vi "WS_Main.vi"(6 "LabVIEW Web Service":refnum<class "Web Service.lvclass">) -> ()   [LabVIEW 2020]
uses:
  <vilib>/wsapi/Web Service.lvclass
  <vilib>/Utility/error.llb/DialogType.ctl
  Libraries/WSsupport/GV_Repos.vi
  Libraries/WSsupport/WSsupport.lvlib
  Libraries/Packages/VIPM/VIPM.lvlib
  Libraries/Packages/GPM/GPM.lvlib
  Libraries/Packages/Packages.lvlib
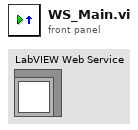
[diagram p1: front panel]
types:
  T1 = typedef "DialogType.ctl" = u16
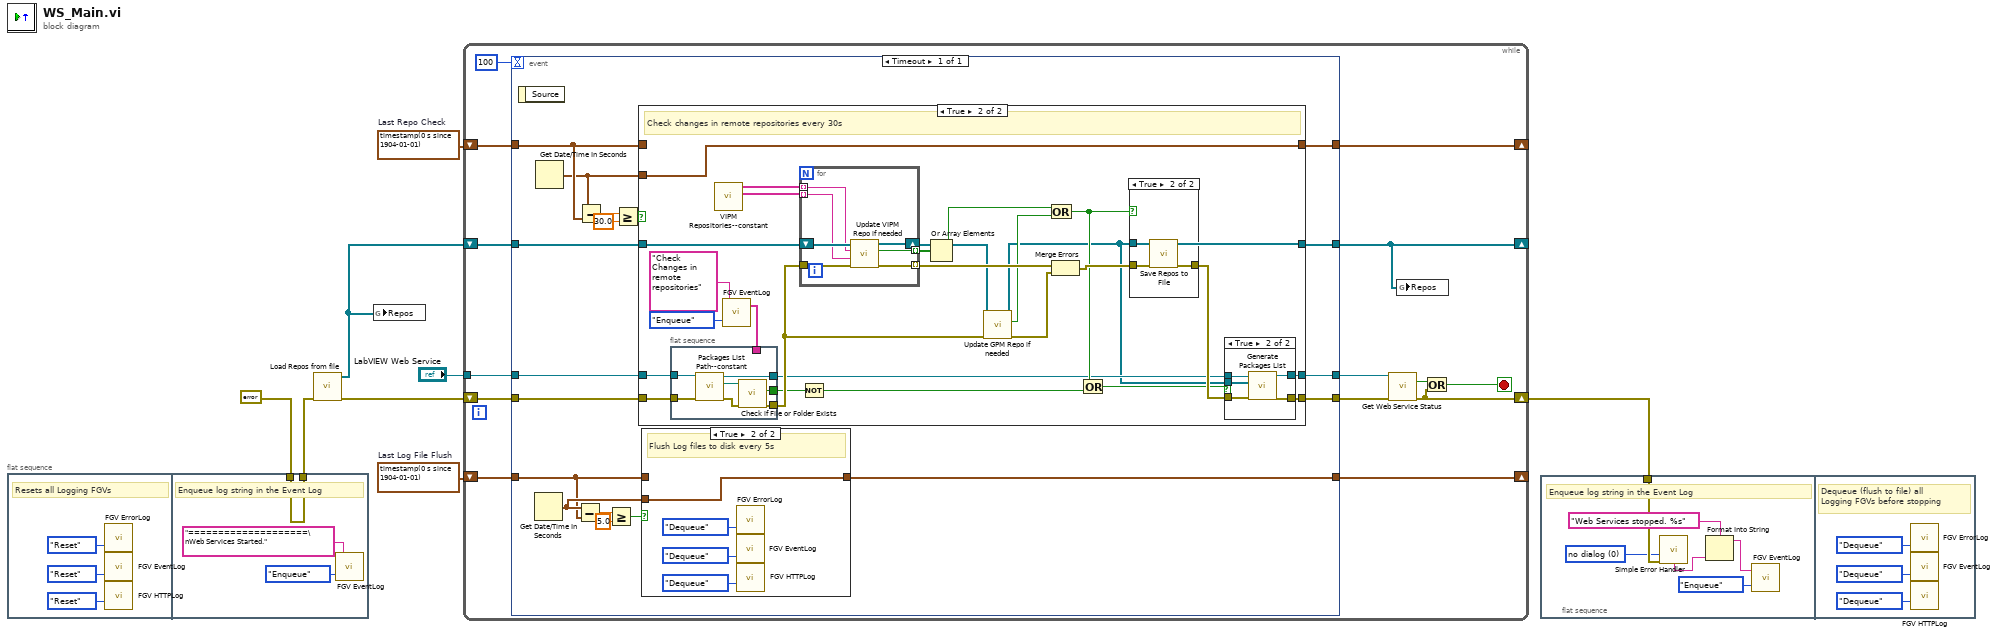
[diagram p0: block diagram]
diagram:
  w2 = timestamp(0 s since 1904-01-01)  # Last Log File Flush
  w7 = timestamp(0 s since 1904-01-01)  # Last Repo Check
  n1 = flat-sequence {
    tunnel: [w14] -> w4
    tunnel: errorcluster {"status"=FALSE, "code"=0, "source"=""} ("error constant") -> [w14]
    frame #0 {
      # "Resets all Logging FGVs"
      n2 = call "FGV ErrorLog.vi"("Action"=enum16{"Reset", "Enqueue", "Dequeue"}."Reset") -> ()  [unwired: 2 in, 1 out]
      n3 = call "FGV EventLog.vi"("Action"=enum16{"Reset", "Enqueue", "Dequeue"}."Reset") -> ()  [unwired: 2 in, 1 out]
      n4 = call "FGV HTTPLog.vi"("Action"=enum16{"Reset", "Enqueue", "Dequeue"}."Reset") -> ()  [unwired: 2 in, 1 out]
    }
    frame #1 {
      # "Enqueue log string in the Event Log"
      n5 = call "FGV EventLog.vi"("Action"=enum16{"Reset", "Enqueue", "Dequeue"}."Enqueue", "String to log"="====================\nWeb Services Started.") -> ()  [unwired: 1 in, 1 out]
    }
  }
  n6 = call "Load Repos from file.vi"("error in"=w4) -> ("error out"=w6:errorcluster, "Repos"=w1:refnum<class "Repo.lvclass">[])  [unwired: 9 in]
  n7 = global write "GV_Repos.vi" "Repos"(w1) -> ()
  n8 = while {
    tunnel: "LabVIEW Web Service" -> [w17]
    shift-right: [w26] -> w3
    shift-left: w6 -> [w20]
    shift-right: [w24] -> _
    shift-left: w7 -> [w23]
    shift-right: [w21] -> _
    shift-left: w1 -> [w22]
    shift-right: [w15] -> _
    shift-left: w2 -> [w16]
    stop <- w27 stop-if-true
    # "Add processing code here. The loop will terminate on error or when the web service stops. If the loop performs long-running operations, consider adding additional Get Web Service Status calls to cancel those operations."
    n9 = event shown="[0] Timeout" {
      selector: _ -> [_]
      dyn-events: _ -> [_]
      timeout: 100 -> [_]
      tunnel: [w39] -> w24
      tunnel: w23 -> [w38]
      tunnel: w22 -> [w43]
      tunnel: [w42] -> w21
      tunnel: [w41] -> w19
      tunnel: w20 -> [w40]
      tunnel: [w36] -> w18
      tunnel: w17 -> [w35]
      tunnel: w16 -> [w30]
      tunnel: [w29] -> w15
      event Timeout {
        n10 = event-data() -> ()  [unwired: 1 in, 1 out]
        n11 = Get Date/Time In Seconds() -> (seconds since 1Jan1904=w31:timestamp)
        n12 = Get Date/Time In Seconds() -> (seconds since 1Jan1904=w37:timestamp)
        n13 = Subtract(x=w31, y=w30) -> (x-y=w34:dbl)
        n14 = Subtract(x=w37, y=w38) -> (x-y=w46:dbl)
        n15 = Greater Or Equal?(x=w34, y=5.0) -> (x >= y?=w32:bool)
        n16 = Greater Or Equal?(x=w46, y=30.0) -> (x >= y?=w44:bool)
        n17 = case shown="True" w44 {
          tunnel: w43 -> [w55 w81]
          tunnel: [w55 w56] -> w42
          tunnel: [w54 w63] -> w41
          tunnel: w40 -> [w54 w73]
          tunnel: [w53 w75] -> w39
          tunnel: w38 -> [w53 _]
          tunnel: w37 -> [_ w75]
          tunnel: [w52 w62] -> w36
          tunnel: w35 -> [w52 w68]
          frame False {
          }
          frame True {
            # "Check changes in remote repositories every 30s"
            n18 = flat-sequence {
              tunnel: w73 -> [w88]
              tunnel: w68 -> [w86]
              tunnel: [w85] -> w67
              tunnel: [w83] -> w66
              tunnel: [w82] -> w61
              tunnel: w57 -> [_]
              frame #0 {
                n19 = call "Packages List Path--constant.vi"("error in (no error)"=w88, "LabVIEW Web Service"=w86) -> ("error out"=w87:errorcluster, "Packages index path"=w84:path, "LabVIEW Web Service out"=w82:refnum<class "Web Service.lvclass">)  [unwired: 7 in]
                n20 = call <vilib>:"Check if File or Folder Exists.vi"("error in (no error)"=w87, "path"=w84) -> ("error out"=w85:errorcluster, "file or folder exists?"=w83:bool)  [unwired: 7 in, 1 out]
              }
            }
            n21 = call "VIPM Repositories--constant.vi"() -> ("Index Filenames"=w69:string[], "Repo URLs"=w70:string[])  [unwired: 10 in]
            n22 = call "FGV EventLog.vi"("Action"=enum16{"Reset", "Enqueue", "Dequeue"}."Enqueue", "String to log"="Check Changes in remote repositories") -> ("Logging"=w57:string[])  [unwired: 1 in]
            n23 = for {
              shift-right: [w105] -> w77
              shift-left: w81 -> [w106]
              tunnel: w70 -> [w104] mode=indexing
              tunnel: [w101] -> w79 mode=indexing
              tunnel: w67 -> [w103]
              tunnel: [w102] -> w80 mode=indexing
              tunnel: w69 -> [w100] mode=indexing
              n24 = call "Update VIPM Repo if needed.vi"("error in (no error)"=w103, "Index filename"=w100, "Repo URL"=w104, "Repos in"=w106) -> ("error out"=w102:errorcluster, "Updated?"=w101:bool, "Repos out"=w105:refnum<class "Repo.lvclass">[])  [unwired: 5 in]
            }
            n25 = Not(x=w66) -> (.not. x?=w65:bool)
            n26 = Or Array Elements(Boolean array=w79) -> (logical OR=w76:bool)
            n27 = call "Update GPM Repo if needed.vi"("error in (no error)"=w67, "Repos in"=w77) -> ("error out"=w72:errorcluster, "Updated?"=w71:bool, "Repos out"=w56:refnum<class "Repo.lvclass">[])  [unwired: 7 in]
            n28 = Compound Arithmetic op=OR(w76, w71) -> (w64:bool)
            n29 = Merge Errors(w80, w72) -> (w74:errorcluster)
            n30 = Or(x=w64, y=w65) -> (x .or. y?=w60:bool)
            n31 = case shown="True" w64 {
              tunnel: w74 -> [w96 w99]
              tunnel: [w96 w97] -> w78
              tunnel: w56 -> [_ w98]
              frame False {
              }
              frame True {
                n32 = call "Save Repos to File.vi"("error in"=w99, "Repos"=w98) -> ("error out"=w97:errorcluster)  [unwired: 8 in, 1 out]
              }
            }
            n33 = case shown="True" w60 {
              tunnel: w78 -> [w89 w95]
              tunnel: [w89 w94] -> w63
              tunnel: [w90 w93] -> w62
              tunnel: w61 -> [w90 w92]
              tunnel: w56 -> [_ w91]
              frame False {
              }
              frame True {
                n34 = call "Generate Packages List.vi"("error in (no error)"=w95, "Repos"=w91, "LabVIEW Web Service"=w92) -> ("error out"=w94:errorcluster, "LabVIEW Web Service out"=w93:refnum<class "Web Service.lvclass">)  [unwired: 7 in]
              }
            }
          }
        }
        n35 = case shown="True" w32 {
          tunnel: [w47 w51] -> w29
          tunnel: w31 -> [_ w51]
          tunnel: w30 -> [w47 _]
          frame False {
          }
          frame True {
            # "Flush Log files to disk every 5s"
            n36 = call "FGV ErrorLog.vi"("Action"=enum16{"Reset", "Enqueue", "Dequeue"}."Dequeue") -> ()  [unwired: 2 in, 1 out]
            n37 = call "FGV EventLog.vi"("Action"=enum16{"Reset", "Enqueue", "Dequeue"}."Dequeue") -> ()  [unwired: 2 in, 1 out]
            n38 = call "FGV HTTPLog.vi"("Action"=enum16{"Reset", "Enqueue", "Dequeue"}."Dequeue") -> ()  [unwired: 2 in, 1 out]
          }
        }
      }
    }
    n39 = call <vilib>:"Get Web Service Status.vi"("LabVIEW Web Service"=w18, "error in (no error)"=w19) -> ("service stopping?"=w28:bool, "error out"=w26:errorcluster)  [unwired: 11 in, 1 out]
    n40 = global write "GV_Repos.vi" "Repos"(w21) -> ()
    n41 = Or(x=w28, y=w26) -> (x .or. y?=w27:bool)
  }
  n42 = flat-sequence {
    tunnel: w3 -> [w112]
    frame #0 {
      w111 = T1 0 items=["no dialog", "OK message", "continue or stop message", "OK message + warnings", "continue/stop + warnings"] ("type of dialog (OK msg:1)")
      # "Enqueue log string in the Event Log"
      n43 = call <vilib>:"Simple Error Handler.vi"("type of dialog (OK msg:1)"=w111, "error in (no error)"=w112) -> ("message"=w109:string)  [unwired: 3 in, 4 out]
      n44 = Format Into String(format string="Web Services stopped. %s", w109) -> (resulting string=w108:string)  [unwired: 2 in, 1 out]
      n45 = call "FGV EventLog.vi"("Action"=enum16{"Reset", "Enqueue", "Dequeue"}."Enqueue", "String to log"=w108) -> ()  [unwired: 1 in, 1 out]
    }
    frame #1 {
      # "Dequeue (flush to file) all Logging FGVs before stopping"
      n46 = call "FGV ErrorLog.vi"("Action"=enum16{"Reset", "Enqueue", "Dequeue"}."Dequeue") -> ()  [unwired: 2 in, 1 out]
      n47 = call "FGV EventLog.vi"("Action"=enum16{"Reset", "Enqueue", "Dequeue"}."Dequeue") -> ()  [unwired: 2 in, 1 out]
      n48 = call "FGV HTTPLog.vi"("Action"=enum16{"Reset", "Enqueue", "Dequeue"}."Dequeue") -> ()  [unwired: 2 in, 1 out]
    }
  }
